vi "Get Headers.vi"(8 "error in (no error)":errorcluster, 11 "Request in":refnum<class "Request.lvclass">) -> (0 "error out":errorcluster, 2 "Headers":cluster{"Header":string, "Value":string}[](array[cluster]), 3 "Request out":refnum<class "Request.lvclass">)   [LabVIEW 2020, in "HTTP Utils.lvlib" / "Request.lvclass"]
uses:
  Request.lvclass
  Request.lvclass/Request.ctl
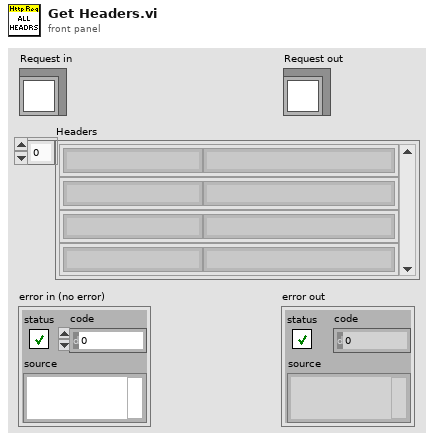
[diagram p1: front panel]
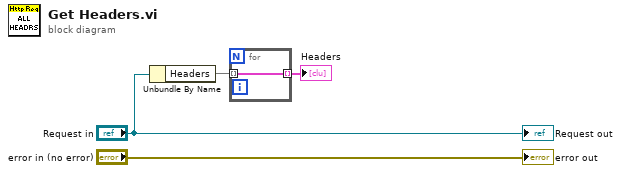
[diagram p0: block diagram]
diagram:
  n1 = Unbundle By Name("Request in") -> ("Headers"=w2:map{string, string})
  n2 = for {
    tunnel: w2 -> [w5] mode=indexing
    tunnel: [w5] -> w1 mode=indexing
  }
  "Headers" <- w1
  "error out" <- "error in (no error)"
  "Request out" <- "Request in"
